vi "Construct Class.vi"(8 "error in (no error)":errorcluster, 10 "Actor in":refnum<class "Engine.lvclass">, 11 "Engine in":refnum<class "Engine.lvclass">) -> (0 "error out":errorcluster, 2 "Actor out":refnum<class "Engine.lvclass">, 3 "Engine out":refnum<class "Engine.lvclass">)   [LabVIEW 2023, in "Engine.lvlib" / "Engine.lvclass"]
uses:
  Library/Engine.lvclass
  Library/Engine.lvclass/Engine.ctl
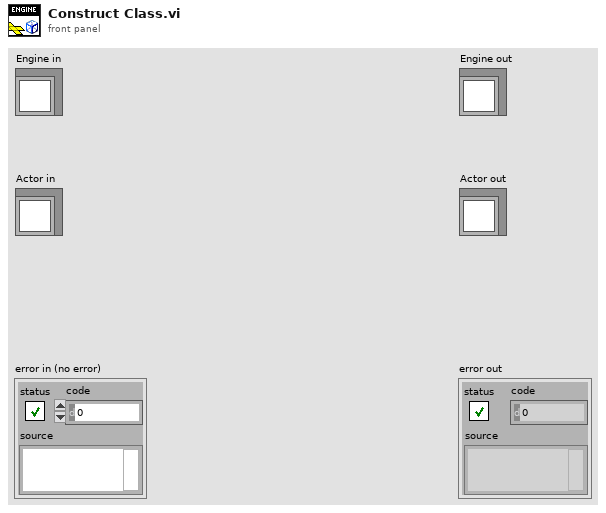
[diagram p1: front panel]
types:
  T1 = typedef "Engine.lvlib/Engine.lvclass/Events.ctl" = cluster{"System":T2, "Other":T3}
  T2 = typedef "Engine.lvlib/Engine.lvclass/SystemEvents.ctl" = cluster{"Fault Monitor":refnum<user-event>, "Status":refnum<user-event>}
  T3 = typedef "Engine.lvlib/Engine.lvclass/OtherEvents.ctl" = cluster{"Launch":refnum<user-event>, "AbstractMessage":refnum<user-event>}
  T4 = typedef "Engine.lvlib/Engine.lvclass/DVRs.ctl" = cluster{"Operator":refnum<data-value>, "Witness":refnum<data-value>, "Model":refnum<data-value>, "Serial":refnum<data-value>, "Pedigree":refnum<data-value>, "TestName":refnum<data-value>}
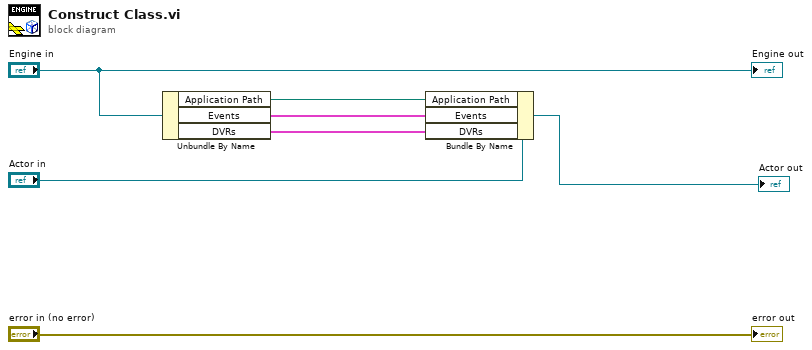
[diagram p0: block diagram]
diagram:
  n1 = Unbundle By Name("Engine in") -> ("Application Path"=w3:path, "Events"=w2:T1, "DVRs"=w1:T4)
  n2 = Bundle By Name(cluster="Actor in", "Application Path"=w3, "Events"=w2, "DVRs"=w1) -> (→"Actor out":refnum<class "Engine.lvclass">)
  "error out" <- "error in (no error)"
  "Engine out" <- "Engine in"
